vi "Deserialize_To_Sibling.vi"(8 "error in (no error)":errorcluster, 10 "To Object":refnum<class>, 11 "From Object":refnum<class>) -> (0 "error out":errorcluster, 3 "Target Object":refnum<class>)   [LabVIEW 2020, in "BlueSerialization.lvlib" / "BlueSerializer.lvclass"]
uses:
  BlueSerializer.lvclass
  <vilib>/Utility/error.llb/Error Cluster From Error Code.vi
  <vilib>/ErrorRing/Error Ring.xnode
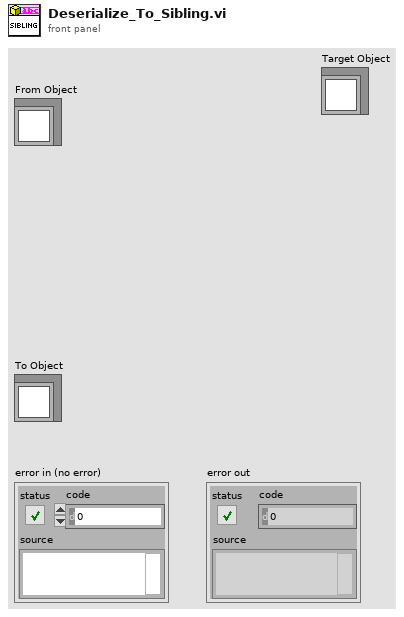
[diagram p1: front panel]
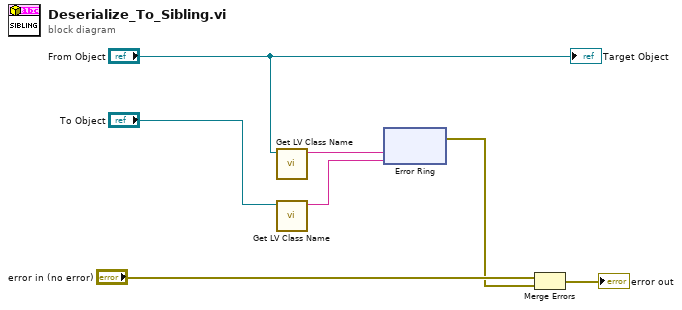
[diagram p0: block diagram]
diagram:
  n1 = call <vilib>:"Get LV Class Name.vi"("object"="From Object") -> ("class name"=w7:string)  [unwired: 9 in, 1 out]
  n2 = call <vilib>:"Get LV Class Name.vi"("object"="To Object") -> ("class name"=w6:string)  [unwired: 9 in, 1 out]
  n3 = xnode "Error Ring"("parameter 0"=w7, "parameter 1"=w6) -> ("error out"=w3:errorcluster)
  n4 = Merge Errors("error in (no error)", w3) -> (→"error out":errorcluster)
  "Target Object" <- "From Object"
